vi "Main.vi"() -> ()   [LabVIEW 2019, in "Setting Panel.lvlib"]
doc: "This template is based off of the Queued Message Handler design pattern and the Queued Message Handler project template that ships with LabVIEW.\n\nThe main difference is that the queue is private to this module and communication between modules is performed via Broadcast and Request events.\n\nRequest events are wrapped in public API methods and are handled in the Event Handling Loop (EHL) of this VI. Any module can register for Broadcast events sent by this module. The EHL generates messages based on user interface actions.\n\nThe Message Handling Loop (MHL) processes messages generated by the EHL, or by other messages. The messages are string values, so new messages can be added easily to the Message Cases case structure in the MHL. Each message cluster can also provide an optional value for Message Data, which is a variant that can be converted to whatever message-specific data is required.\n_____\nBased on Delacor QMH Project Template 4.2.1.64."
uses:
  Setting Panel.lvlib
  <vilib>/Delacor/Delacor QMH/Libraries/Module Admin_class/Delacor_lib_QMH_Module Admin.lvclass
  TypeDef/ISO.ctl
  TypeDef/Noise.ctl
  Module Data--cluster.ctl
  Do Something Argument--cluster.ctl
  <vilib>/Delacor/Delacor QMH/Libraries/Message Queue_class/Delacor_lib_QMH_Message Queue.lvclass/Delacor_lib_QMH_Message Queue.ctl
  Do Something Else Argument--cluster.ctl
  Do Something Else and Wait for Reply Argument--cluster.ctl
  Do Something Else and Wait (Reply Payload)--cluster.ctl
  Stop Argument--cluster.ctl
  <vilib>/Delacor/Delacor QMH/Libraries/Module Admin_class/Delacor_lib_QMH_Module Admin.lvclass/Delacor_lib_QMH_Module Admin.ctl
  <vilib>/Utility/miscctls.llb/LVPointTypeDef.ctl
  TypeDef/Sett data.ctl
  TypeDef/Link.ctl
  <vilib>/Delacor/Delacor QMH/Libraries/Message Queue_class/Delacor_lib_QMH_Enqueue Message (Single).vi
  <vilib>/Delacor/Delacor QMH/Libraries/Module Admin_class/Delacor_lib_QMH_Get External Launch.vi
  <vilib>/Utility/error.llb/Error Cluster From Error Code.vi
  <vilib>/ErrorRing/Error Ring.xnode
  <vilib>/Delacor/Delacor QMH/Libraries/Message Queue_class/Delacor_lib_QMH_Message Queue.lvclass
panel:
  out "Tab Control":enum32{"Public settings", "Private settings"}(tab)
  in  "Максимальная дистанция":dbl
  in  "Максимальный уровень шума":dbl
  in  "Apply":bool
  out "Скорость":dbl=4.0 min=4.0 max=128.0 step=4.0
  out "Порядок фильтра":i32=4 min=4 max=128 step=4
  out "Усилитель":dbl=4.0 min=4.0 max=128.0 step=4.0
  in  "ISO/IEC":T1
  out "M":cluster{"Метка":i64, "Считыветель":i64}={"Метка"=4, "Считыветель"=4} {"Считыветель" min=4 max=128 step=4; "Метка" min=4 max=128 step=4}
  out "БУПУЭМСМ":cluster{"R":dbl, "C":dbl, "L":dbl} {"L" format="%#_6p"; "C" format="%#_6p"; "R" format="%#_6p"}
  out "БУПУЭМСС":cluster{"R":dbl, "C":dbl, "L":dbl} {"L" format="%#_6p"; "C" format="%#_6p"; "R" format="%#_6p"}
  out "Type noise":T2
  in  "Type noise w":T2
  in  "M w":cluster{"Метка":i64, "Считыветель":i64}={"Метка"=10, "Считыветель"=10} {"Считыветель" min=10 max=10 step=100; "Метка" min=10 max=10 step=100}
  in  "BM":cluster{"R":dbl, "C":dbl, "L":dbl}={"R"=1.0, "C"=0.01, "L"=1e-05} {"L" min=1e-05 max=1.5e-05 step=1e-06 format="%#_6p"; "C" min=0.01 max=0.15 step=0.001 format="%#_6p"; "R" min=1.0 max=150.0 step=1.0 format="%#_6p"}
  in  "BI":cluster{"R":dbl, "C":dbl, "L":dbl}={"R"=1.0, "C"=0.01, "L"=1e-05} {"L" min=1e-05 max=1.5e-05 step=1e-06 format="%#_6p"; "C" min=0.01 max=0.15 step=0.001 format="%#_6p"; "R" min=1.0 max=150.0 step=1.0 format="%#_6p"}
  in  "Write":bool
  in  "ISO/IEC w":T1
  in  "Bit rate":dbl=4.0 min=4.0 max=128.0 step=4.0
  in  "Gain":dbl=4.0 min=1.0 max=100.0 step=1.0
  in  "Filter":i32=4 min=1 max=15 step=1
  in  "Simulate MHL Error":bool
  in  "Simulate EHL Error":bool
  out "error out":errorcluster
  in  "Module Admin":refnum<class "Delacor_lib_QMH_Module Admin.lvclass">
  out "X":dbl
  out "Status":string
  in  "Do Something Else <Replace Me>":bool
  in  "Do Something <Replace Me>":bool
  # "Коэффициент модуляции, %"
  # "Коэффициент модуляции, %"
  # "БУПУЭМСС"
  # "Коэфициент скорости"
  # "Усилитель"
  # "БУПУЭМСМ"
  # "Порядок фильтра"
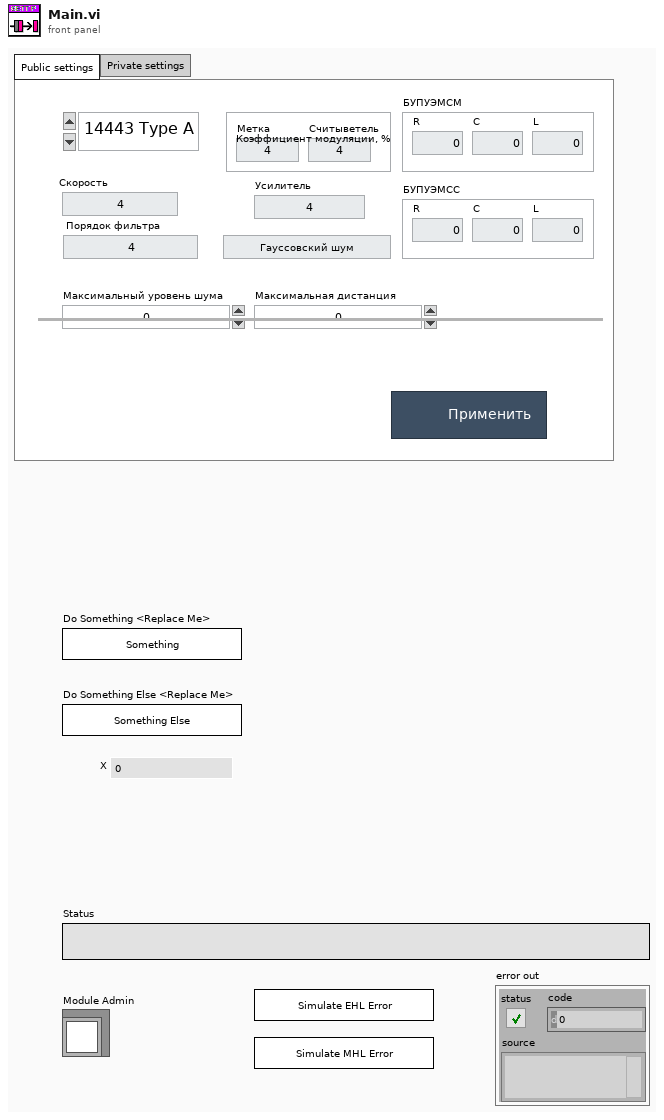
[diagram p1: front panel]
types:
  T1 = typedef "ISO.ctl" = enum16{"14443 Type A", "14443 Type B", "Felica", "15693"}
  T2 = typedef "Noise.ctl" = enum16{"Гауссовский шум", "Белый шум"}
  T3 = typedef "Setting Panel.lvlib/Request Events--cluster.ctl" = cluster{"Stop Module":refnum<user-event>, "Do Something":refnum<user-event>, "Do Something Else":refnum<user-event>, "Do Something Else and Wait for Reply":refnum<user-event>, "Show Panel":refnum<user-event>, "Hide Panel":refnum<user-event>, "Get Module Execution Status":refnum<user-event>, "Show Diagram":refnum<user-event>}
  T4 = typedef "Setting Panel.lvlib/Module Data--cluster.ctl" = cluster{"Status":string}
  T5 = typedef "Setting Panel.lvlib/Do Something Argument--cluster.ctl" = cluster{"Do Something Msg":string}
  T6 = typedef "Setting Panel.lvlib/Do Something Else Argument--cluster.ctl" = cluster{"Do Something Else Msg":string, "X":dbl}
  T7 = typedef "Setting Panel.lvlib/Do Something Else and Wait for Reply Argument--cluster.ctl" = cluster{"Do Something Else Msg":string, "X":dbl, "Wait Notifier":refnum<notifier>, "wait for reply":bool}
  T8 = enum32{"invalid lock state", "Not Locked", "Locked (No Password)", "Password-protected"}
  T9 = typedef "Setting Panel.lvlib/Stop Argument--cluster.ctl" = cluster{"Origin":string, "Exit via Stop Module Req?":bool, "Wait for Module to stop?":bool}
  T10 = typedef "LVPointTypeDef.ctl" = cluster{"Horizontal":i16, "Vertical":i16}
  T11 = enum32{"Invalid", "Standard", "Closed", "Hidden", "Minimized", "Maximized"}
  T12 = typedef "Setting Panel.lvlib/Do Something Else and Wait (Reply Payload)--cluster.ctl" = cluster{"Value":dbl, "error":errorcluster}
  T13 = typedef "Sett data.ctl" = cluster{"Filter":i32, "Gain":dbl, "Bit rate":dbl, "ISO/IEC w ":T1, "BI":cluster{"R":dbl, "C":dbl, "L":dbl}, "BM":cluster{"R":dbl, "C":dbl, "L":dbl}, "M":cluster{"Метка":i64, "Считыветель":i64}, "Type noise":T2, "Link":T14, "Noise attenuator":dbl, "Signal gain":dbl, "Distance":dbl}
  T14 = typedef "Link.ctl" = enum16{"UPLINK", "DOWNLINK"}
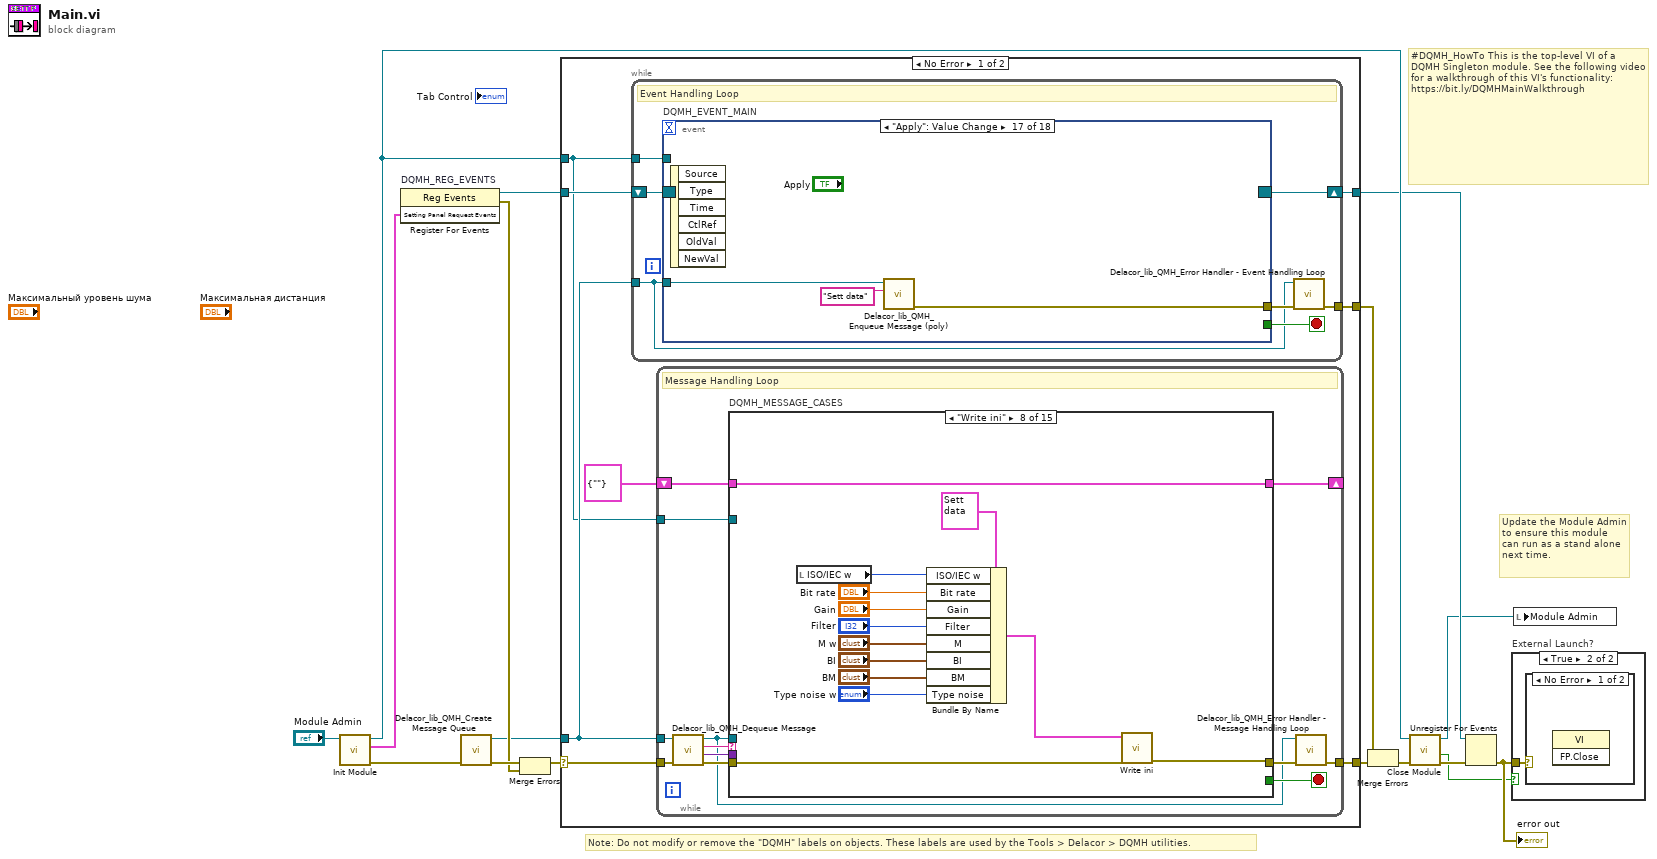
[diagram p0: block diagram]
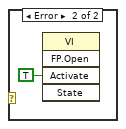
[diagram p3: hidden frame]
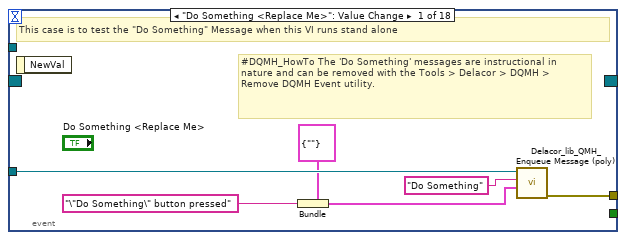
[diagram p4: hidden frame]
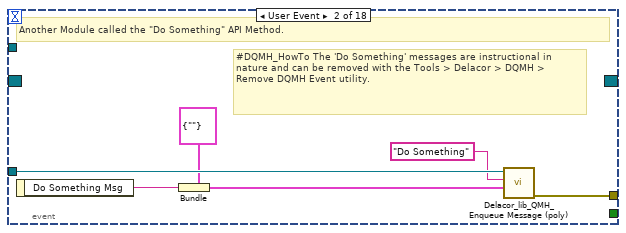
[diagram p5: hidden frame]
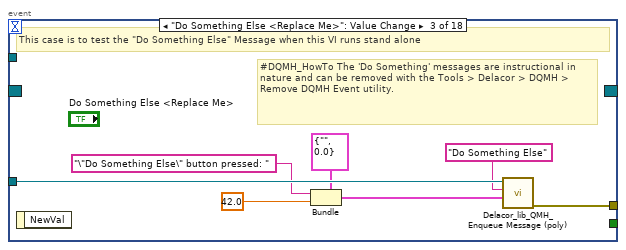
[diagram p6: hidden frame]
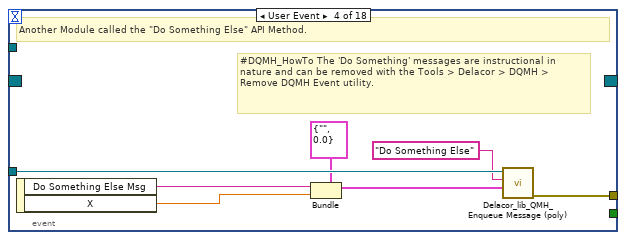
[diagram p7: hidden frame]
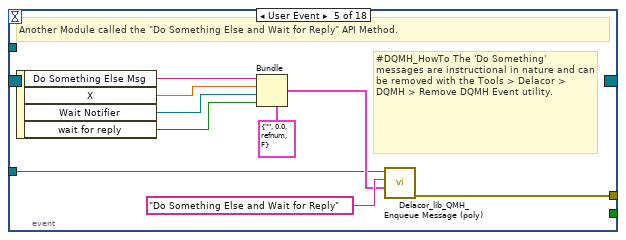
[diagram p8: hidden frame]
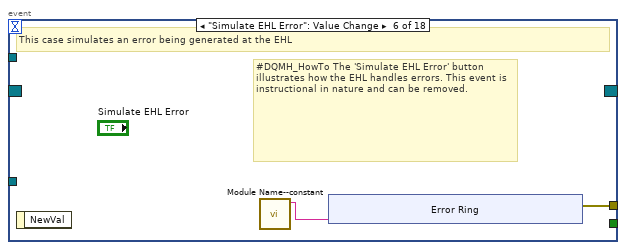
[diagram p9: hidden frame]
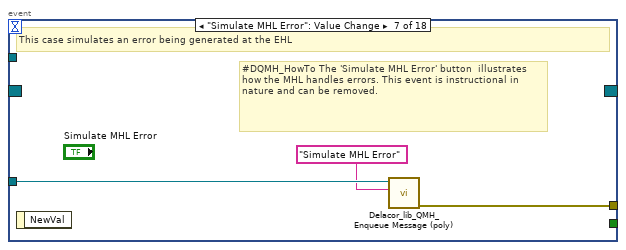
[diagram p10: hidden frame]
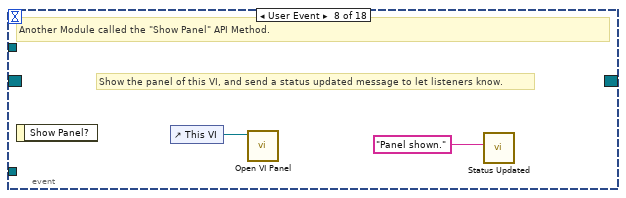
[diagram p11: hidden frame]
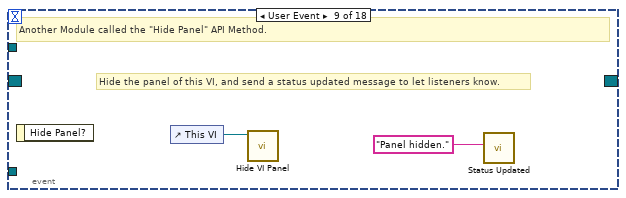
[diagram p12: hidden frame]
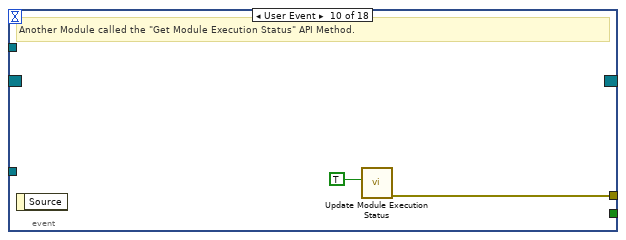
[diagram p13: hidden frame]
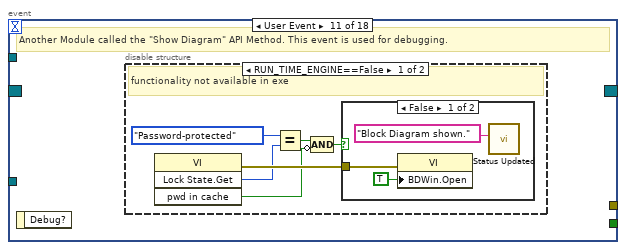
[diagram p14: hidden frame]
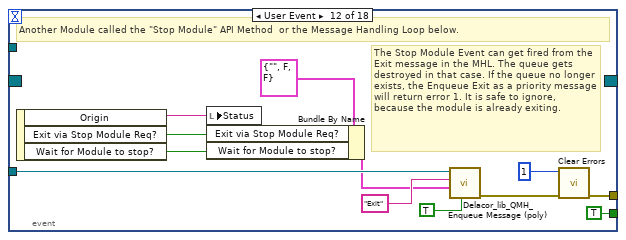
[diagram p17: hidden frame]
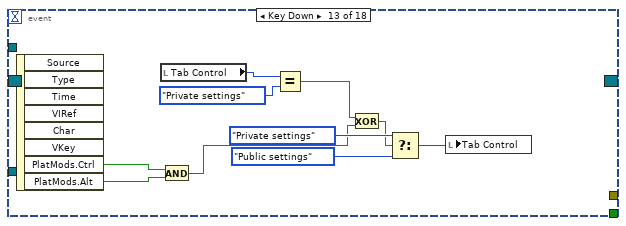
[diagram p18: hidden frame]
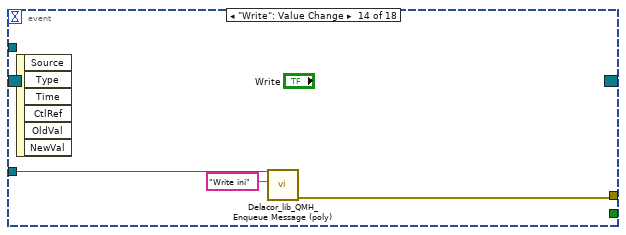
[diagram p19: hidden frame]
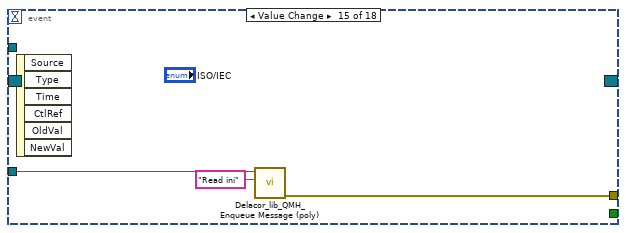
[diagram p20: hidden frame]
diagram:
  # "#DQMH_HowTo This is the top-level VI of a DQMH Singleton module. See the following video for a walkthrough of this VI's functionality: https://bit.ly/DQMHMainWalkthrough"
  # "Note: Do not modify or remove the \"DQMH\" labels on objects. These labels are used by the Tools > Delacor > DQMH utilities."
  # "Update the Module Admin to ensure this module can run as a stand alone next time."
  n1 = call "Init Module.vi"("Singleton Module Admin in"="Module Admin") -> ("error out"=w16:errorcluster, "Setting Panel Request Events"=w5:T3, "Singleton Module Admin out"=w8:refnum<class "Delacor_lib_QMH_Module Admin.lvclass">)  [unwired: 8 in]
  n2 = register-events "DQMH_REG_EVENTS"(w5) -> (reference out=w6:refnum<event-registration>, error out=w9:errorcluster)  [unwired: 2 in]
  n3 = call <vilib>:"Delacor_lib_QMH_Create Message Queue.vi"("error in (no error)"=w16) -> ("error out"=w11:errorcluster, "Message Queue"=w4:refnum<class "Delacor_lib_QMH_Message Queue.lvclass">)  [unwired: 9 in]
  n4 = Merge Errors(w11, w9) -> (w10:errorcluster)
  n5 = case shown="No Error" w10 {
    selector: w10 -> [w23 w349]
    tunnel: [w25 w349] -> w17
    tunnel: [w22 w346] -> w7
    tunnel: w6 -> [w20 w346]
    tunnel: w4 -> [w19 _]
    tunnel: [w24 _] -> w14
    tunnel: w8 -> [w18 w342]
    frame No Error {
      n6 = while {
        tunnel: w19 -> [w26]
        shift-right: [w29] -> w22
        shift-left: w20 -> [w30]
        tunnel: [w31] -> w24
        tunnel: w18 -> [w27]
        stop <- w28 stop-if-true
        # "Event Handling Loop"
        n7 = event "DQMH_EVENT_MAIN" shown="[16] \"Apply\": Value Change" {
          selector: w30 -> [_ _ _ _ _ _ _ _ _ _ _ _ _ _ _ _ _ _]
          dyn-events: [_ _ _ _ _ _ _ _ _ _ _ _ _ _ _ _ _ _] -> w29
          timeout: _ -> [_ _ _ _ _ _ _ _ _ _ _ _ _ _ _ _ _ _]
          tunnel: [_ _ _ _ _ _ _ _ _ _ _ TRUE ("Discard?") _ _ _ _ _ _] -> w28
          tunnel: w26 -> [w37 w43 w50 w57 w60 _ w78 _ _ _ _ w102 _ w118 w121 w124 w127 w131]
          tunnel: [w38 w44 w51 w58 w67 w69 w79 _ _ w85 _ w105 _ w119 w120 w123 w126 w133] -> w32
          tunnel: w27 -> [_ _ _ _ _ _ _ _ _ _ _ _ _ _ _ _ _ w130]
          event "Do Something <Replace Me>": Value Change {
            # "#DQMH_HowTo The 'Do Something' messages are instructional in nature and can be removed with the Tools > Delacor > DQMH > Remove DQMH Event utility."
            # "This case is to test the \"Do Something\" Message when this VI runs stand alone"
            n8 = event-data() -> ()  [unwired: 1 in, 1 out]
            n9 = Bundle(cluster=T5 {"Do Something Msg"=""} ("Do Something Argument"), "Do Something Msg"="\"Do Something\" button pressed" ("\"Do Something\" button pressed")) -> (w33:T5)
            n10 = call-poly <vilib>:"Delacor_lib_QMH_Enqueue Message (poly).vi"("Message Data"=w33, "Message"="Do Something", "Message Queue in"=w37) -> ("error out"=w38:errorcluster)  [unwired: 7 in, 1 out]
          }
          event User Event {
            # "#DQMH_HowTo The 'Do Something' messages are instructional in nature and can be removed with the Tools > Delacor > DQMH > Remove DQMH Event utility."
            # "Another Module called the \"Do Something\" API Method."
            n11 = event-data() -> ("Do Something Msg"=w40:string)  [unwired: 1 in]
            n12 = Bundle(cluster=T5 {"Do Something Msg"=""} ("Do Something Argument"), "Do Something Msg"=w40) -> (w39:T5)
            n13 = call-poly <vilib>:"Delacor_lib_QMH_Enqueue Message (poly).vi"("Message Data"=w39, "Message"="Do Something", "Message Queue in"=w43) -> ("error out"=w44:errorcluster)  [unwired: 7 in, 1 out]
          }
          event "Do Something Else <Replace Me>": Value Change {
            # "#DQMH_HowTo The 'Do Something' messages are instructional in nature and can be removed with the Tools > Delacor > DQMH > Remove DQMH Event utility."
            # "This case is to test the \"Do Something Else\" Message when this VI runs stand alone"
            n14 = event-data() -> ()  [unwired: 1 in, 1 out]
            n15 = Bundle(cluster=T6 {"Do Something Else Msg"="", "X"=0.0} ("Do Something Else Argument"), "Do Something Else Msg"="\"Do Something Else\" button pressed: " ("\"Do Something Else\" button pressed"), "X"=42.0) -> (w47:T6)
            n16 = call-poly <vilib>:"Delacor_lib_QMH_Enqueue Message (poly).vi"("Message Data"=w47, "Message"="Do Something Else", "Message Queue in"=w50) -> ("error out"=w51:errorcluster)  [unwired: 7 in, 1 out]
          }
          event User Event {
            # "#DQMH_HowTo The 'Do Something' messages are instructional in nature and can be removed with the Tools > Delacor > DQMH > Remove DQMH Event utility."
            # "Another Module called the \"Do Something Else\" API Method."
            n17 = event-data() -> ("Do Something Else Msg"=w53:string, "X"=w52:dbl)  [unwired: 1 in]
            n18 = Bundle(cluster=T6 {"Do Something Else Msg"="", "X"=0.0} ("Do Something Else Argument"), "Do Something Else Msg"=w53, "X"=w52) -> (w54:T6)
            n19 = call-poly <vilib>:"Delacor_lib_QMH_Enqueue Message (poly).vi"("Message Data"=w54, "Message"="Do Something Else", "Message Queue in"=w57) -> ("error out"=w58:errorcluster)  [unwired: 7 in, 1 out]
          }
          event User Event {
            # "#DQMH_HowTo The 'Do Something' messages are instructional in nature and can be removed with the Tools > Delacor > DQMH > Remove DQMH Event utility."
            # "Another Module called the \"Do Something Else and Wait for Reply\" API Method."
            n20 = event-data() -> ("Do Something Else Msg"=w63:string, "X"=w62:dbl, "Wait Notifier"=w61:refnum<notifier>, "wait for reply"=w59:bool)  [unwired: 1 in]
            n21 = Bundle(cluster=T7 {"Do Something Else Msg"="", "X"=0.0, "Wait Notifier"=refnum, "wait for reply"=FALSE} ("Do Something Else and Wait for Reply Argument"), "Do Something Else Msg"=w63, "X"=w62, "Wait Notifier"=w61, "wait for reply"=w59) -> (w64:T7)
            n22 = call-poly <vilib>:"Delacor_lib_QMH_Enqueue Message (poly).vi"("Message Data"=w64, "Message"="Do Something Else and Wait for Reply", "Message Queue in"=w60) -> ("error out"=w67:errorcluster)  [unwired: 7 in, 1 out]
          }
          event "Simulate EHL Error": Value Change {
            # "#DQMH_HowTo The 'Simulate EHL Error' button  illustrates how the EHL handles errors. This event is instructional in nature and can be removed."
            # "This case simulates an error being generated at the EHL"
            n23 = event-data() -> ()  [unwired: 1 in, 1 out]
            n24 = call "Module Name--constant.vi"() -> ("Module Name"=w68:string)  [unwired: 11 in]
            n25 = xnode "Error Ring"("parameter 0"=w68) -> ("error out"=w69:errorcluster)
          }
          event "Simulate MHL Error": Value Change {
            # "#DQMH_HowTo The 'Simulate MHL Error' button  illustrates how the MHL handles errors. This event is instructional in nature and can be removed."
            # "This case simulates an error being generated at the EHL"
            n26 = event-data() -> ()  [unwired: 1 in, 1 out]
            n27 = call-poly <vilib>:"Delacor_lib_QMH_Enqueue Message (poly).vi"("Message"="Simulate MHL Error", "Message Queue in"=w78) -> ("error out"=w79:errorcluster)  [unwired: 8 in, 1 out]
          }
          event User Event {
            # "Show the panel of this VI, and send a status updated message to let listeners know."
            # "Another Module called the \"Show Panel\" API Method."
            n28 = event-data() -> ()  [unwired: 1 in, 1 out]
            n29 = control-ref of="This VI"() -> (w81:refnum<vi>)
            n30 = call "Open VI Panel.vi"("VI"=w81) -> ()  [unwired: 10 in, 1 out]
            n31 = call "Status Updated.vi"("Status"="Panel shown." ("format string")) -> ()  [unwired: 10 in, 1 out]
          }
          event User Event {
            # "Hide the panel of this VI, and send a status updated message to let listeners know."
            # "Another Module called the \"Hide Panel\" API Method."
            n32 = event-data() -> ()  [unwired: 1 in, 1 out]
            n33 = control-ref of="This VI"() -> (w83:refnum<vi>)
            n34 = call "Hide VI Panel.vi"("VI"=w83) -> ()  [unwired: 10 in, 1 out]
            n35 = call "Status Updated.vi"("Status"="Panel hidden." ("format string")) -> ()  [unwired: 10 in, 1 out]
          }
          event User Event {
            # "Another Module called the \"Get Module Execution Status\" API Method."
            n36 = event-data() -> ()  [unwired: 1 in, 1 out]
            n37 = call "Update Module Execution Status.vi"("Running?"=TRUE) -> ("error out"=w85:errorcluster)  [unwired: 10 in]
          }
          event User Event {
            # "Another Module called the \"Show Diagram\" API Method. This event is used for debugging."
            n38 = event-data() -> ()  [unwired: 1 in, 1 out]
            n39 = disable-structure shown="RUN_TIME_ENGINE==False" {
              frame condition #0 (active) {
                # "functionality not available in exe"
                n40 = invoke class="VI" method="Lock State.Get"() -> (error out=w91:errorcluster, "Get Lock State"=w90:T8, "pwd in cache"=w87:bool)  [unwired: 4 in, 1 out]
                n41 = Equal?(x=T8."Password-protected", y=w90) -> (x = y?=w88:bool)
                n42 = Compound Arithmetic op=AND(w88, invert w87) -> (w86:bool)
                n43 = case shown="False" w86 {
                  tunnel: w91 -> [w94 _]
                  frame False {
                    n44 = property class="VI"(error in=w94, "BDWin.Open"=TRUE ("Block Diagram Window:Open")) -> ()  [unwired: 1 in, 2 out]
                    n45 = call "Status Updated.vi"("Status"="Block Diagram shown." ("format string")) -> ()  [unwired: 10 in, 1 out]
                  }
                  frame True {
                    # "Password-protected VI, and the password is not in the cache. Do not show the diagram."
                  }
                }
              }
              frame condition #1 {
              }
            }
          }
          event User Event {
            # "The Stop Module Event can get fired from the Exit message in the MHL. The queue gets destroyed in that case. If the queue no longer exists, the Enqueue Exit as a priority message will return error 1. It is safe to ignore, because the module is already exiting."
            # "Another Module called the \"Stop Module\" API Method  or the Message Handling Loop below."
            n46 = event-data() -> ("Origin"=w101:string, "Exit via Stop Module Req?"=w97:bool, "Wait for Module to stop?"=w96:bool)  [unwired: 1 in]
            n47 = local write "Status"(w101) -> ()
            n48 = Bundle By Name(cluster=T9 {"Origin"="", "Exit via Stop Module Req?"=FALSE, "Wait for Module to stop?"=FALSE} ("Stop Argument"), "Exit via Stop Module Req?"=w97, "Wait for Module to stop?"=w96) -> (w95:T9)
            n49 = call-poly <vilib>:"Delacor_lib_QMH_Enqueue Message (poly).vi"("Priority Message? (F)"=TRUE, "Message Data"=w95, "Message"="Exit", "Message Queue in"=w102) -> ("error out"=w106:errorcluster)  [unwired: 6 in, 1 out]
            n50 = call <vilib>:"Clear Errors.vi"("error in (no error)"=w106, "specific error code to clear (0: all)"=1) -> ("error out"=w105:errorcluster)  [unwired: 4 in, 1 out]
          }
          event Key Down {
            n51 = event-data() -> ("PlatMods.Ctrl"=w114:bool, "PlatMods.Alt"=w115:bool)  [unwired: 1 in, 6 out]
            n52 = local read "Tab Control"() -> (w111:enum32{"Public settings", "Private settings"})
            n53 = And(x=w114, y=w115) -> (x .and. y?=w109:bool)
            n54 = Equal?(x=w111, y=enum32{"Public settings", "Private settings"}."Private settings" ("Tab Control")) -> (x = y?=w108:bool)
            n55 = Exclusive Or(1:w109, 2:w108) -> (0:w107:bool)
            n56 = Select(t=enum32{"Public settings", "Private settings"}."Private settings" ("Tab Control"), s=w107, f=enum32{"Public settings", "Private settings"}."Public settings" ("Tab Control")) -> (s? t:f=w112:enum32{"Public settings", "Private settings"})
            n57 = local write "Tab Control"(w112) -> ()
          }
          event "Write": Value Change {
            n58 = event-data() -> ()  [unwired: 1 in, 6 out]
            n59 = call-poly <vilib>:"Delacor_lib_QMH_Enqueue Message (poly).vi"("Message"="Write ini", "Message Queue in"=w118) -> ("error out"=w119:errorcluster)  [unwired: 8 in, 1 out]
          }
          event Value Change {
            n60 = event-data() -> ()  [unwired: 1 in, 6 out]
            n61 = call-poly <vilib>:"Delacor_lib_QMH_Enqueue Message (poly).vi"("Message"="Read ini", "Message Queue in"=w121) -> ("error out"=w120:errorcluster)  [unwired: 8 in, 1 out]
          }
          event Value Change {
            n62 = event-data() -> ()  [unwired: 1 in, 6 out]
            n63 = call-poly <vilib>:"Delacor_lib_QMH_Enqueue Message (poly).vi"("Message"="Read ini write", "Message Queue in"=w124) -> ("error out"=w123:errorcluster)  [unwired: 8 in, 1 out]
          }
          event "Apply": Value Change {
            n64 = event-data() -> ()  [unwired: 1 in, 6 out]
            n65 = call-poly <vilib>:"Delacor_lib_QMH_Enqueue Message (poly).vi"("Message"="Sett data", "Message Queue in"=w127) -> ("error out"=w126:errorcluster)  [unwired: 8 in, 1 out]
          }
          event Panel Close? {
            w132 = TRUE  # Discard the event, the MHL is responsible for closing and stopping this VI.
            # "Hide the panel or send the 'Exit' message if the user clicks the 'X' on the module main VI panel."
            n66 = event-data() -> ()  [unwired: 1 in, 1 out]
            n67 = property class="Module Admin"(reference=w130) -> ("Accessors:External Launch"=w129:bool)  [unwired: 1 in, 2 out]
            n68 = case shown="True" w129 {
              tunnel: w131 -> [_ w137]
              tunnel: [_ w138] -> w133
              frame True {
                # "If externally launched, clicking the 'X' hides the panel, but doesn't close it."
                n69 = control-ref of="This VI"() -> (w134:refnum<vi>)
                n70 = call "Hide VI Panel.vi"("VI"=w134) -> ()  [unwired: 10 in, 1 out]
              }
              frame False {
                # "If run as a stand-alone VI, clicking the panel 'X' stops the VI."
                n71 = call-poly <vilib>:"Delacor_lib_QMH_Enqueue Message (poly).vi"("Priority Message? (F)"=TRUE, "Message"="Exit", "Message Queue in"=w137) -> ("error out"=w138:errorcluster)  [unwired: 7 in, 1 out]
              }
            }
            n72 = event-data("Discard?"=w132) -> ()  [unwired: 1 in, 1 out]
          }
        }
        n73 = call-dynamic "Delacor_lib_QMH_Error Handler - Event Handling Loop.vi"("error in (no error)"=w32, "Message Queue in"=w26) -> ("dup error in"=w31:errorcluster)  [unwired: 8 in, 1 out]
      }
      n74 = while {
        tunnel: w19 -> [w141]
        shift-right: [w145] -> _
        shift-left: T4 {"Status"=""} ("Data Cluster") -> [w146]
        tunnel: w23 -> [w149]
        tunnel: [w147] -> w25
        tunnel: w18 -> [w139]
        stop <- w144 stop-if-true
        # "Message Handling Loop"
        n75 = call-dynamic "Delacor_lib_QMH_Dequeue Message.vi"("error in (no error)"=w149, "Message Queue in"=w141) -> ("error out"=w148:errorcluster, "Message Data"=w142:variant, "Message"=w143:string, "Message Queue out"=w140:refnum<class "Delacor_lib_QMH_Message Queue.lvclass">)  [unwired: 6 in]
        n76 = case "DQMH_MESSAGE_CASES" shown="\"Write ini\"" w143 {
          selector: w143 -> [_ _ _ _ _ _ _ _ _ _ _ _ _ _ w329]
          tunnel: w140 -> [w152 _ _ _ _ _ _ _ _ _ _ _ w299 w321 _]
          tunnel: w148 -> [w172 w176 w184 w193 w212 w227 w239 w251 w267 w277 w284 w289 w306 w327 w331]
          tunnel: [w171 w176 w182 w192 w211 w226 w238 w250 w266 w269 w284 w288 w302 w324 w332] -> w150
          tunnel: w146 -> [w162 w175 w181 w191 w209 w225 w241 w254 w268 w282 w283 w286 w301 w320 w330]
          tunnel: [w161 w175 w181 w191 w209 w225 w241 w254 w268 w282 w283 w286 w301 w320 w330] -> w145
          tunnel: [_ _ _ _ _ _ _ _ _ _ _ _ _ w319 _] -> w144
          tunnel: w142 -> [_ _ w180 w188 w206 _ _ _ _ _ _ _ w300 w318 _]
          tunnel: w139 -> [w163 _ _ _ _ _ _ _ _ _ _ _ w298 w313 _]
          frame "Initialize" {
            w156 = "Initial Message" ("Initial Message")
            # "Initialize - Any operation that needs to be done before the module can receive messages. Synchronize Caller Events.vi will inform Start Module.vi that the module has launched and is ready to receive messages. Module Did Init.vi will broadcast that the module initialized."
            n77 = call "Synchronize Caller Events.vi"("error in (no error)"=w172, "Singleton Module Admin in"=w163) -> ("error out"=w154:errorcluster, "Singleton Module Admin out"=w158:refnum<class "Delacor_lib_QMH_Module Admin.lvclass">)  [unwired: 8 in]
            n78 = property class="Module Admin"(reference=w158) -> ("Accessors:External Launch"=w167:bool)  [unwired: 1 in, 2 out]
            n79 = call-poly <vilib>:"Delacor_lib_QMH_Enqueue Message (poly).vi"("error in (no error)"=w154, "Message"="Read ini", "Message Queue in"=w152) -> ("error out"=w153:errorcluster)  [unwired: 7 in, 1 out]
            n80 = local write "Tab Control"(enum32{"Public settings", "Private settings"}."Public settings" ("Tab Control")) -> ()
            n81 = Select(t=T11."Hidden" ("State"), s=w167, f=T11."Standard" ("State")) -> (s? t:f=w164:T11)
            n82 = call "Module Name--constant.vi"() -> ("Module Name"=w170:string)  [unwired: 11 in]
            n83 = property class="VI"("Front Panel.Title"=w170) -> (reference out=w169:refnum<vi>, error out=w174:errorcluster)  [unwired: 2 in]
            n84 = call "Module Name--constant.vi"() -> ("Module Name"=w159:string)  [unwired: 11 in]
            n85 = invoke class="VI" method="FP.Open"(reference=w169, error in=w174, "State"=w164) -> (reference out=w168:refnum<vi>, error out=w173:errorcluster)  [unwired: 2 in, 3 out]
            n86 = Bundle By Name(cluster=w162, "Status"=w156) -> (w161:T4)
            n87 = call "Module Did Init.vi"("error in (no error)"=w153, "Initialized?"=TRUE, "Origin"=w159) -> ("error out"=w171:errorcluster)  [unwired: 8 in]
            n88 = invoke class="VI" method="FP.Center"(reference=w168, error in=w173) -> ()  [unwired: 1 in, 3 out]
            n89 = property on="Pane" class="Pane"("Origin"=T10 {"Horizontal"=0, "Vertical"=0}) -> ()  [unwired: 2 in, 2 out]
            "Status" <- w156
          }
          frame "--- Module Specific ---" {
            # "Separator -- The following cases handle messages specific to this Module."
          }
          frame "Do Something" {
            # "#DQMH_HowTo The 'Do Something' messages are instructional in nature and can be removed with the Tools > Delacor > DQMH > Remove DQMH Event utility."
            # "Do Something - Replace this message with functionality for your own application. Note that this message also fires the \"Did Something\" broadcast event."
            n90 = Variant To Data(error in=w184, type=T5 {"Do Something Msg"=""} ("Do Something Argument"), Variant=w180) -> (data=w179:T5, error out=w183:errorcluster)
            n91 = Unbundle By Name(w179) -> ("Do Something Msg"=w177:string)
            n92 = call "Did Something.vi"("error in (no error)"=w183, "Did Something Msg"=w177) -> ("error out"=w182:errorcluster)  [unwired: 9 in]
            n93 = local write "Status"(w177) -> ()
            n94 = call "Status Updated.vi"("Status"=w177) -> ()  [unwired: 10 in, 1 out]
          }
          frame "Do Something Else" {
            # "#DQMH_HowTo The 'Do Something' messages are instructional in nature and can be removed with the Tools > Delacor > DQMH > Remove DQMH Event utility."
            # "Do Something Else - Replace this message with functionality for your own application."
            n95 = Variant To Data(error in=w193, type=T6 {"Do Something Else Msg"="", "X"=0.0} ("Do Something Else Argument"), Variant=w188) -> (data=w189:T6, error out=w192:errorcluster)
            n96 = Unbundle By Name(w189) -> ("Do Something Else Msg"=w187:string, "X"=w186:dbl)
            "X" <- w186
            n97 = Format Into String(initial string=w187, w186) -> (resulting string=w185:string)  [unwired: 2 in, 1 out]
            n98 = local write "Status"(w185) -> ()
            n99 = call "Status Updated.vi"("Status"=w185) -> ()  [unwired: 10 in, 1 out]
          }
          frame "Do Something Else and Wait for Reply" {
            w201 = "X(%.2f)+Offset(%.2f)=%.2f"  # status message format string
            # "#DQMH_HowTo The 'Do Something' messages are instructional in nature and can be removed."
            # "Send back X with a random offset"
            # "Do Something Else and Wait for Reply - Replace this message with functionality for your own application. Note that this message must fire a notifier to let callers know it has finished execution, and it returns an error if the 'Value' is negative."
            n100 = Random Number (0-1)() -> (number: 0 to 1=w203:dbl)
            n101 = Variant To Data(error in=w212, type=T7 {"Do Something Else Msg"="", "X"=0.0, "Wait Notifier"=refnum, "wait for reply"=FALSE} ("Do Something Else and Wait for Reply Argument"), Variant=w206) -> (data=w207:T7, error out=w210:errorcluster)
            n102 = Unbundle By Name(w207) -> ("Wait Notifier"=w194:refnum<notifier>, "Do Something Else Msg"=w205:string, "X"=w202:dbl, "wait for reply"=w198:bool)
            n103 = Add(x=w203, y=w202) -> (x+y=w197:dbl)
            n104 = local write "X"(w202) -> ()
            n105 = Less Than 0?(x=w197) -> (x < 0?=w200:bool)
            n106 = Format Into String(format string=w201, initial string=w205, w202, w203, w197) -> (resulting string=w199:string)  [unwired: 1 in, 1 out]
            n107 = case shown="True" w200 {
              tunnel: [_ w219] -> w195
              frame False {
              }
              frame True {
                n108 = xnode "Error Ring"() -> ("error out"=w219:errorcluster)
              }
            }
            n109 = Bundle By Name(cluster=T12 {"Value"=0.0, "error"={"status"=FALSE, "code"=0, "source"=""}} ("notification"), "error"=w195, "Value"=w197) -> (w196:T12)
            n110 = local write "Status"(w199) -> ()
            n111 = call "Status Updated.vi"("Status"=w199) -> ()  [unwired: 10 in, 1 out]
            n112 = case shown="True" w198 {
              tunnel: w196 -> [_ w215]
              tunnel: w194 -> [_ w214]
              frame False {
              }
              frame True {
                # "Simulate an operation that requires a wait."
                n113 = flat-sequence {
                  tunnel: w215 -> [w218]
                  tunnel: w214 -> [w217]
                  tunnel: w213 -> [_]
                  frame #0 {
                    n114 = Send Notification(notification=w218, notifier=w217) -> ()  [unwired: 1 in, 2 out]
                  }
                }
                n115 = Wait (ms)(milliseconds to wait=u32 1000) -> (millisecond timer value=w213:u32)
              }
            }
            n116 = Merge Errors(w210, w195) -> (w211:errorcluster)
          }
          frame "---Copy This Frame---" {
            # "Duplicate this frame when creating new messages.  Change this comment in the duplicated frame to describe this message."
            n117 = Merge Errors(w227) -> (w226:errorcluster)
          }
          frame "Sett data" {
            n118 = local read "БУПУЭМСМ"() -> (w230:cluster{"R":dbl, "C":dbl, "L":dbl})
            n119 = local read "БУПУЭМСС"() -> (w231:cluster{"R":dbl, "C":dbl, "L":dbl})
            n120 = local read "Усилитель"() -> (w234:dbl)
            n121 = local read "Type noise"() -> (w228:T2)
            n122 = local read "Скорость"() -> (w233:dbl)
            n123 = local read "ISO/IEC"() -> (w232:T1)
            n124 = local read "Filter"() -> (w235:i32)
            n125 = local read "M"() -> (w229:cluster{"Метка":i64, "Считыветель":i64})
            n126 = Bundle By Name(cluster=T13 {"Filter"=0, "Gain"=0.0, "Bit rate"=0.0, "ISO/IEC w "=enum."14443 Type A", "BI"={"R"=0.0, "C"=0.0, "L"=0.0}, "BM"={"R"=0.0, "C"=0.0, "L"=0.0}, "M"={"Метка"=4, "Считыветель"=4}, "Type noise"=enum."Гауссовский шум", "Link"=enum."UPLINK", "Noise attenuator"=0.0, "Signal gain"=1.0, "Distance"=0.0} ("Sett data"), "Filter"=w235, "Gain"=w234, "Bit rate"=w233, "ISO/IEC w"=w232, "BI"=w231, "BM"=w230, "M"=w229, "Type noise"=w228) -> (w237:T13)
            n127 = To Variant(anything=w237) -> (Variant=w236:variant)
            n128 = call "Get data.vi"("error in (no error)"=w239, "Variant"=w236) -> ("error out"=w238:errorcluster)  [unwired: 9 in]
          }
          frame "Write ini" {
            n129 = local read "ISO/IEC w"() -> (w242:T1)
            n130 = Bundle By Name(cluster=T13 {"Filter"=0, "Gain"=0.0, "Bit rate"=0.0, "ISO/IEC w "=enum."14443 Type A", "BI"={"R"=0.0, "C"=0.0, "L"=0.0}, "BM"={"R"=0.0, "C"=0.0, "L"=0.0}, "M"={"Метка"=4, "Считыветель"=4}, "Type noise"=enum."Гауссовский шум", "Link"=enum."UPLINK", "Noise attenuator"=0.0, "Signal gain"=1.0, "Distance"=0.0} ("Sett data"), "ISO/IEC w"=w242, "Bit rate"="Bit rate", "Gain"="Gain", "Filter"="Filter", "M"="M w", "BI"="BI", "BM"="BM", "Type noise"="Type noise w") -> (w252:T13)
            n131 = call "Write ini.vi"("error in (no error)"=w251, "Sett data"=w252) -> ("error out"=w250:errorcluster)  [unwired: 9 in]
          }
          frame "Read ini" {
            n132 = local read "ISO/IEC"() -> (w262:T1)
            n133 = Bundle By Name(cluster=T13 {"Filter"=0, "Gain"=0.0, "Bit rate"=0.0, "ISO/IEC w "=enum."14443 Type A", "BI"={"R"=0.0, "C"=0.0, "L"=0.0}, "BM"={"R"=0.0, "C"=0.0, "L"=0.0}, "M"={"Метка"=4, "Считыветель"=4}, "Type noise"=enum."Гауссовский шум", "Link"=enum."UPLINK", "Noise attenuator"=0.0, "Signal gain"=1.0, "Distance"=0.0} ("Sett data"), "ISO/IEC w"=w262) -> (w264:T13)
            n134 = call "Read ini.vi"("error in (no error)"=w267, "Sett data"=w264) -> ("error out"=w266:errorcluster, "Sett data out"=w263:T13)  [unwired: 8 in]
            n135 = Unbundle By Name(w263) -> ("Bit rate"=→"Скорость":dbl, "Gain"=→"Усилитель":dbl, "Filter"=→"Порядок фильтра":i32, "M"=→"M":cluster{"Метка":i64, "Считыветель":i64}, "BM"=→"БУПУЭМСМ":cluster{"R":dbl, "C":dbl, "L":dbl}, "BI"=→"БУПУЭМСС":cluster{"R":dbl, "C":dbl, "L":dbl}, "Type noise"=→"Type noise":T2)
          }
          frame "Read ini write" {
            n136 = local read "ISO/IEC w"() -> (w279:T1)
            n137 = Bundle By Name(cluster=T13 {"Filter"=0, "Gain"=0.0, "Bit rate"=0.0, "ISO/IEC w "=enum."14443 Type A", "BI"={"R"=0.0, "C"=0.0, "L"=0.0}, "BM"={"R"=0.0, "C"=0.0, "L"=0.0}, "M"={"Метка"=4, "Считыветель"=4}, "Type noise"=enum."Гауссовский шум", "Link"=enum."UPLINK", "Noise attenuator"=0.0, "Signal gain"=1.0, "Distance"=0.0} ("Sett data"), "ISO/IEC w"=w279) -> (w281:T13)
            n138 = call "Read ini.vi"("error in (no error)"=w277, "Sett data"=w281) -> ("error out"=w269:errorcluster, "Sett data out"=w280:T13)  [unwired: 8 in]
            n139 = Unbundle By Name(w280) -> ("Bit rate"=w276:dbl, "Gain"=w275:dbl, "Filter"=w274:i32, "M"=w273:cluster{"Метка":i64, "Считыветель":i64}, "BM"=w272:cluster{"R":dbl, "C":dbl, "L":dbl}, "BI"=w271:cluster{"R":dbl, "C":dbl, "L":dbl}, "Type noise"=w270:T2)
            n140 = local write "Gain"(w275) -> ()
            n141 = local write "Bit rate"(w276) -> ()
            n142 = local write "Filter"(w274) -> ()
            n143 = local write "M w"(w273) -> ()
            n144 = local write "BM"(w272) -> ()
            n145 = local write "BI"(w271) -> ()
            n146 = local write "Type noise w"(w270) -> ()
          }
          frame "--- Exit and Error Handling---" {
            # "Separator - The following cases handle errors and exit messages."
          }
          frame "Simulate MHL Error" {
            # "#DQMH_HowTo The 'Simulate MHL Error' button  illustrates how the MHL handles errors. This event is instructional in nature and can be removed."
            # "Simulate an error occurring at the MHL"
            n147 = call "Module Name--constant.vi"() -> ("Module Name"=w285:string)  [unwired: 11 in]
            n148 = xnode "Error Ring"("parameter 0"=w285) -> ("error out"=w287:errorcluster)
            n149 = Merge Errors(w289, w287) -> (w288:errorcluster)
          }
          frame "Error" {
            # "#CodeRecommended - If you ever change the name of this \"Error\" message, you'll need to update the name in the Check Loop Error.vi as well."
            # "#CodeRecommended - If the module is running in standalone mode (External Launch = FALSE), this code will pop up an error dialog and call the 'Exit' message if an error occurs. Add more fine-grained error handling here."
            # "Error - Check the error message data and respond accordingly. This message is sent by the \"Error Handler\" VIs at the end of each loop in this application."
            n150 = property class="Module Admin"(reference=w298) -> ("Accessors:External Launch"=w297:bool)  [unwired: 1 in, 2 out]
            n151 = Variant To Data(error in=w306, type=errorcluster {"status"=FALSE, "code"=0, "source"=""} ("error constant"), Variant=w300) -> (data=w307:errorcluster, error out=w304:errorcluster)
            n152 = call "Error Reported.vi"("Error"=w307) -> ()  [unwired: 10 in, 1 out]
            n153 = case shown="False" w297 {
              tunnel: [w312 _] -> w303
              tunnel: w299 -> [w310 _]
              tunnel: w307 -> [w311 _]
              frame False {
                # "If the module is running standalone, then pop up an error dialog and call the \"Exit\" message."
                n154 = call <vilib>:"Simple Error Handler.vi"("error in (no error)"=w311) -> ()  [unwired: 4 in, 5 out]
                n155 = call-poly <vilib>:"Delacor_lib_QMH_Enqueue Message (poly).vi"("Priority Message? (F)"=TRUE, "Message"="Exit", "Message Queue in"=w310) -> ("error out"=w312:errorcluster)  [unwired: 7 in, 1 out]
              }
              frame True {
                # "If the module was launched externally, calling the Error Reported broadcast VI is the only action performed by the \"Error\" message. The module's caller can then process the error appropriately."
              }
            }
            n156 = Merge Errors(w304, w303) -> (w302:errorcluster)
            n157 = local write "error out"(w302) -> ()
          }
          frame "Exit" {
            w317 = 91  # 91: not all Exit messages will have an argument
            w319 = TRUE  # Stop the VI
            # "Release the message queue reference"
            # "#CodeNeeded - Add any required cleanup code here"
            # "Exit - Exit the application."
            n158 = Variant To Data(error in=w327, type=T9 {"Origin"="", "Exit via Stop Module Req?"=FALSE, "Wait for Module to stop?"=FALSE} ("Stop Argument"), Variant=w318) -> (data=w315:T9, error out=w323:errorcluster)
            n159 = call <vilib>:"Clear Errors.vi"("error in (no error)"=w323, "specific error code to clear (0: all)"=w317) -> ("error out"=w326:errorcluster)  [unwired: 4 in, 1 out]
            n160 = control-ref of="This VI"() -> (w314:refnum<vi>)
            n161 = call-dynamic "Delacor_lib_QMH_Release Message Queue.vi"("error in (no error)"=w326, "Message Queue"=w321) -> ("error out"=w325:errorcluster)  [unwired: 9 in]
            n162 = call "Handle Exit.vi"("Stop Argument"=w315, "Admin in"=w313, "VI reference"=w314) -> ("error out"=w322:errorcluster)  [unwired: 7 in, 1 out]
            n163 = Merge Errors(w325, w322) -> (w324:errorcluster)
          }
          frame Default {
            # "'Default' case only runs if there is a message that isn't defined in any of the other cases.  Output a programming error."
            n164 = call "Module Name--constant.vi"() -> ("Module Name"=w328:string)  [unwired: 11 in]
            n165 = xnode "Error Ring"("parameter 0"=w329, "parameter 1"=w328) -> ("error out"=w333:errorcluster)
            n166 = Merge Errors(w331, w333) -> (w332:errorcluster)
          }
        }
        n167 = call-dynamic "Delacor_lib_QMH_Error Handler - Message Handling Loop.vi"("error in (no error)"=w150, "Message Queue in"=w140) -> ("dup error in"=w147:errorcluster)  [unwired: 8 in, 1 out]
      }
    }
    frame Error {
      # "Synchronize Caller Events.vi will inform Start Module.vi that the module has launched and will let the code calling Start Module.vi register for broadcasts and would permit the caller receive the broadcast that an error occurred at launch time."
      n168 = call "Synchronize Caller Events.vi"("Singleton Module Admin in"=w342) -> ("error out"=w347:errorcluster)  [unwired: 9 in, 1 out]
      n169 = call "Module Name--constant.vi"() -> ("Module Name"=w345:string)  [unwired: 11 in]
      n170 = Format Into String(format string="An error occurred during initialization. %s is no longer running.", w345) -> (resulting string=w343:string)  [unwired: 2 in, 1 out]
      n171 = Merge Errors(w349, w347) -> (w348:errorcluster)
      n172 = call "Error Reported.vi"("Additional Information"=w343, "Error"=w348) -> ()  [unwired: 9 in, 1 out]
    }
  }
  n173 = Merge Errors(w14, w17) -> (w13:errorcluster)
  n174 = call "Close Module.vi"("error in (no error)"=w13, "Module Admin in"=w8) -> ("error out"=w15:errorcluster, "External Launch"=w1:bool, "Module Admin out"=w2:refnum<class "Delacor_lib_QMH_Module Admin.lvclass">)  [unwired: 7 in]
  n175 = Unregister For Events(event registration refnum=w7, error in=w15) -> (error out=w12:errorcluster)
  "error out" <- w12
  n176 = case "External Launch?" shown="True" w1 {
    tunnel: w12 -> [_ w350]
    frame False {
    }
    frame True {
      n177 = case shown="No Error" w350 {
        frame No Error {
          n178 = invoke class="VI" method="FP.Close"() -> ()  [unwired: 3 in, 3 out]
        }
        frame Error {
          n179 = invoke class="VI" method="FP.Open"("Activate"=TRUE ("Activate?")) -> ()  [unwired: 4 in, 5 out]
        }
      }
    }
  }
  n180 = local write "Module Admin"(w2) -> ()
